vi "Calculate Winning Vote.vi"(11 "Vote Count":T1[](array[typedef])) -> (3 "Vote":string)   [LabVIEW 2019]
uses:
  Vote Result.ctl
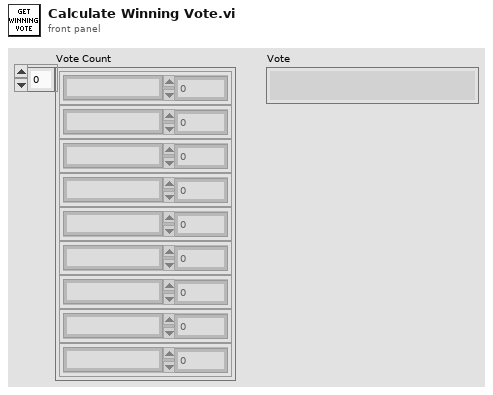
[diagram p1: front panel]
types:
  T1 = typedef "Vote Result.ctl" = cluster{"Vote":string, "Count":i32}
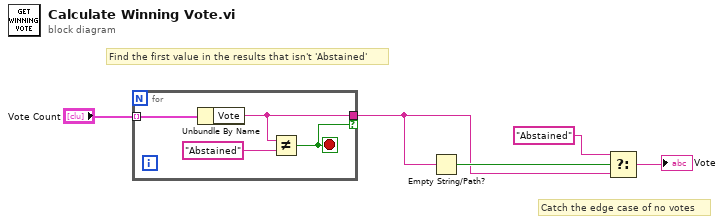
[diagram p0: block diagram]
diagram:
  # "Catch the edge case of no votes"
  # "Find the first value in the results that isn't 'Abstained'"
  n1 = for {
    tunnel: "Vote Count" -> [w9] mode=indexing
    tunnel: [w7] -> w2 if=w6
    stop <- w6 stop-if-true
    n2 = Unbundle By Name(w9) -> ("Vote"=w7:string)
    n3 = Not Equal?(x=w7, y="Abstained") -> (x != y?=w6:bool)
  }
  n4 = Empty String/Path?(string/path=w2) -> (empty?=w4:bool)
  n5 = Select(t="Abstained" ("y"), s=w4, f=w2) -> (s? t:f=→"Vote":string)
